vi "grafica.vi"() -> ()   [LabVIEW 2020]
panel:
  out "Waveform Graph":dynamicdata(graph)
  in  "stop":bool
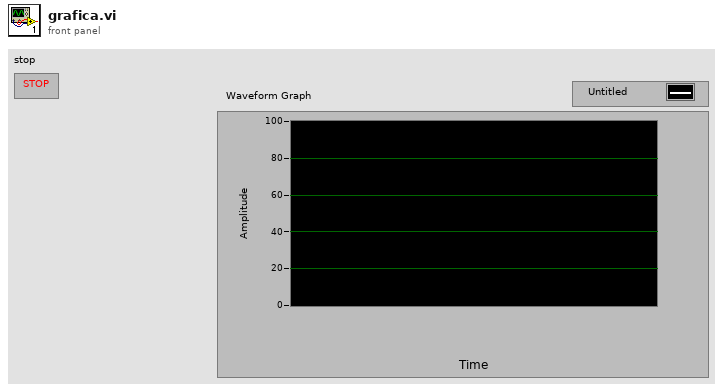
[diagram p1: front panel]
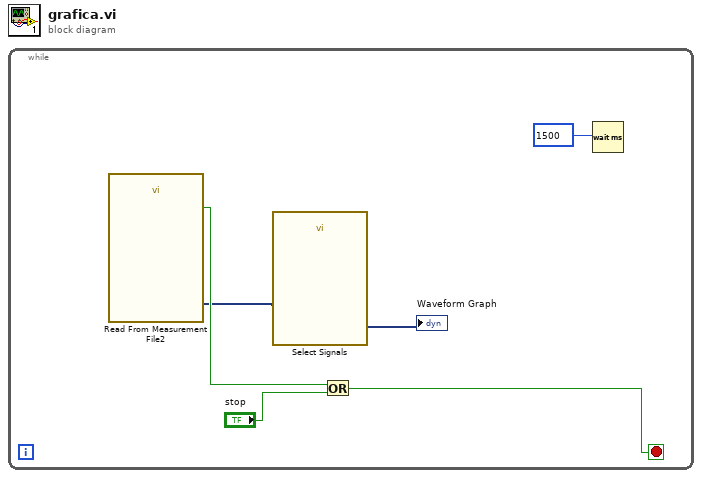
[diagram p0: block diagram]
diagram:
  n1 = while {
    stop <- w4 stop-if-true
    n2 = call "Read From Measurement File2"() -> ("Signals"=w2:dynamicdata, "EOF?"=w5:bool)  [unwired: 6 in, 4 out]
    n3 = call "Select Signals"("Signals"=w2) -> ("Signal Out"=→"Waveform Graph":dynamicdata)  [unwired: 9 in, 1 out]
    n4 = Or(x=w5, y="stop") -> (x .or. y?=w4:bool)
    n5 = Wait (ms)(milliseconds to wait=1500) -> ()  [unwired: 1 out]
  }
